vi "stringAddCTRT.vi"(3 "string":string) -> (1 "strOut":string)   [LabVIEW 2012]
doc: "This VI add Return/lineFeed"
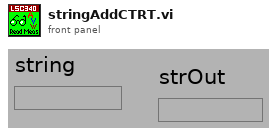
[diagram p1: front panel]
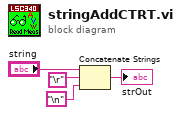
[diagram p0: block diagram]
diagram:
  n1 = Concatenate Strings("string", "\r", "\n") -> (→"strOut":string)
